vi "Settings Dialog.vi"(8 "error in (no error)":errorcluster, 11 "Feed Module Config in":T15={"GUID"="", "Drop Coords"={"Horizontal"=0, "Vertical"=0}, "Process Name"="", "Settings"={"Cycle Period"=500.0, "Ismatech"={"VISA resource name"="", "Simulated?"=TRUE, "Pump Number"=1.0, "Reverse?"=FALSE}, "Masterflex"={"VISA resource name"="", "Simulated?"=TRUE, "Pump Number"=1.0, "Reverse?"=FALSE}, "Mettler"={"VISA resource name"="", "Simulated?"=FALSE}, "Bronkhorst M13 Flow Meter"={"VISA resource name"="", "Simulated?"=TRUE}, "PID 2 Parameters"={"Input Device"=enum."Default", "Output Device"=enum."Default", "Setpoint"=0.0, "PID gains"={"proportional gain (Kc)"=1.0, "integral time (Ti, min)"=0.01, "derivative time (Td, min)"=0.0}}, "Manual Entry"=0.0, "Auto?"=TRUE, "output range"={"output high"=100.0, "output low"=0.0}, "Bronkhorst M14"={"VISA resource name"="", "Simulated?"=FALSE}, "Tacmina Settings"={"Analog DAQ Task"="", "Digital DAQ Task"=""}, "KNF SIMDOS Settings"={"VISA resource name"="", "Simulated?"=TRUE}, "ASIA Pump C"={"ASIA Pump #"=-1, "channel"=-1, "Simulated"=FALSE}, "VICI Settings"={"VISA resource name"="", "Simulated?"=TRUE, "Pump Letter"="", "Reverse?"=FALSE}, "FLOM Settings"={"VISA resource name"="", "Simulated?"=TRUE, "Pump Number"=0.0}, "SSI PR Settings"={"VISA resource name"="", "Simulated?"=FALSE}}, "Settings Load Count"=0, "OP Load Count"=0} {"Settings"."output range"."output low" min=0.0 max=100.0 format="%.2f"; "Settings"."output range"."output high" format="%.2f"; "Settings"."PID 2 Parameters"."PID gains"."derivative time (Td, min)" format="%.3f"; "Settings"."PID 2 Parameters"."PID gains"."integral time (Ti, min)" format="%.3f"; "Settings"."PID 2 Parameters"."PID gains"."proportional gain (Kc)" format="%.3f"; "Settings"."ASIA Pump C"."channel" min=0 max=1 step=1; "Settings"."Ismatech"."Pump Number" min=1.0 max=20.0 step=1.0; "Settings"."Masterflex"."Pump Number" min=1.0 max=20.0 step=1.0}) -> (0 "error out":errorcluster, 1 "Cancelled?":bool=TRUE, 2 "UI Refresh Needed?":bool, 3 "Feed Module Config out":T15={"GUID"="", "Drop Coords"={"Horizontal"=0, "Vertical"=0}, "Process Name"="", "Settings"={"Cycle Period"=500.0, "Ismatech"={"VISA resource name"="", "Simulated?"=TRUE, "Pump Number"=1.0, "Reverse?"=FALSE}, "Masterflex"={"VISA resource name"="", "Simulated?"=TRUE, "Pump Number"=1.0, "Reverse?"=FALSE}, "Mettler"={"VISA resource name"="", "Simulated?"=FALSE}, "Bronkhorst M13 Flow Meter"={"VISA resource name"="", "Simulated?"=TRUE}, "PID 2 Parameters"={"Input Device"=enum."Default", "Output Device"=enum."Default", "Setpoint"=0.0, "PID gains"={"proportional gain (Kc)"=1.0, "integral time (Ti, min)"=0.01, "derivative time (Td, min)"=0.0}}, "Manual Entry"=0.0, "Auto?"=TRUE, "output range"={"output high"=100.0, "output low"=0.0}, "Bronkhorst M14"={"VISA resource name"="", "Simulated?"=FALSE}, "Tacmina Settings"={"Analog DAQ Task"="", "Digital DAQ Task"=""}, "KNF SIMDOS Settings"={"VISA resource name"="", "Simulated?"=TRUE}, "ASIA Pump C"={"ASIA Pump #"=0, "channel"=0, "Simulated"=FALSE}, "VICI Settings"={"VISA resource name"="", "Simulated?"=TRUE, "Pump Letter"="", "Reverse?"=FALSE}, "FLOM Settings"={"VISA resource name"="", "Simulated?"=TRUE, "Pump Number"=0.0}, "SSI PR Settings"={"VISA resource name"="", "Simulated?"=FALSE}}, "Settings Load Count"=0, "OP Load Count"=0} {"Settings"."output range"."output low" min=0.0 max=100.0 format="%.2f"; "Settings"."output range"."output high" format="%.2f"; "Settings"."PID 2 Parameters"."PID gains"."derivative time (Td, min)" format="%.3f"; "Settings"."PID 2 Parameters"."PID gains"."integral time (Ti, min)" format="%.3f"; "Settings"."PID 2 Parameters"."PID gains"."proportional gain (Kc)" format="%.3f"; "Settings"."ASIA Pump C"."channel" min=0 max=1 step=1; "Settings"."Ismatech"."Pump Number" min=1.0 max=20.0 step=1.0; "Settings"."Masterflex"."Pump Number" min=1.0 max=20.0 step=1.0})   [LabVIEW 2018, in "Feed Module.lvlib" / "Settings.lvlib"]
doc: "Dialog for selecting user specified settings."
uses:
  Settings.lvlib
  Feed Module/Controls/Feed Module Config Cluster.ctl
  <vilib>/Utility/miscctls.llb/LVPoint32TypeDef.ctl
  Feed Module/Controls/Feed Module Settings Cluster.ctl
  Ismatec ISM 831C/Controls/Ismatech Settings Cluster.ctl
  Masterflex 7550-30/Controls/Settings Cluster.ctl
  Mettler Toledo/Controls/Settings Cluster.ctl
  Bronkhorst M13 Flow Meter/Settings Cluster.ctl
  Measure Instrument/PID 2 Parameters Cluster.ctl
  Measure Instrument/PID Input Enum.ctl
  Measure Instrument/PID 2 Output Enum.ctl
  Tacmina QI/Tacmina QI DAQ Setting.ctl
  KNF Pump/Settings Cluster plus SIMDOS.ctl
  ASIA Pump/Pump Settings.ctl
  VICI M50 Party Mode/Settings Cluster.ctl
  FLOM Pump/Settings Cluster.ctl
  SSI PR Class/SSI PR Settings Cluster.ctl
  Bronkhorst M14 Flow Meter/Settings Cluster.ctl
  Ismatec ISM 831C/Ismatec ISM 831C.lvlib
  Masterflex 7550-30/Masterflex 7550-30.lvlib
  Mettler Toledo/Mettler Toledo.lvlib
  Bronkhorst M13 Flow Meter/Bronkhorst M13 Flow Meter.lvlib
  Bronkhorst M14 Flow Meter/Bronkhorst M14 Flow Meter.lvlib
  KNF Pump/KNF SIMDOS.lvlib
  VICI M50 Party Mode/VICI M6 M50 Party Mode.lvlib
  FLOM Pump/FLOM Pump.lvlib
  ASIA Pump.lvlib
  SSI PR Class/SSI PR Pump.lvlib
  <vilib>/Utility/xml.llb/Write to XML File(string).vi
  Feed Module/Feed Module.lvlib
  Tacmina QI/Tacmina QI.lvlib
panel:
  in  "Module Name":string
  in  "Settings Dialog":T14={"Cycle Period"=500.0, "Ismatech"={"VISA resource name"="", "Simulated?"=FALSE, "Pump Number"=1.0, "Reverse?"=FALSE}, "Masterflex"={"VISA resource name"="", "Simulated?"=FALSE, "Pump Number"=1.0, "Reverse?"=FALSE}, "Mettler"={"VISA resource name"="", "Simulated?"=FALSE}, "Bronkhorst M13 Flow Meter"={"VISA resource name"="", "Simulated?"=FALSE}, "PID 2 Parameters"={"Input Device"=enum."Default", "Output Device"=enum."Default", "PID gains"={"proportional gain (Kc)"=1.0, "integral time (Ti, min)"=0.01, "derivative time (Td, min)"=0.0}}, "PID2 Range"={"output high"=100.0, "output low"=0.0}, "Bronkhorst M14 Settings"={"VISA resource name"="", "Simulated?"=FALSE}, "Tacmina Settings"={"Analog DAQ Task"="", "Digital DAQ Task"=""}, "KNF SIMDOS Settings"={"VISA resource name"="", "Simulated?"=FALSE}, "ASIA Pump C"={"ASIA Pump #"=-1, "channel"=-1, "Simulated"=FALSE}, "VICI M50 Settings"={"VISA resource name"="", "Simulated?"=FALSE, "Pump Letter"="", "Reverse?"=FALSE}, "FLOM Settings"={"VISA resource name"="", "Simulated?"=FALSE, "Pump Number"=1.0}, "SSI PR Settings"={"VISA resource name"="", "Simulated?"=FALSE}} {"ASIA Pump C"."channel" min=-1 max=1 step=1; "PID2 Range"."output low" min=0.0 max=100.0 format="%.2f"; "PID2 Range"."output high" format="%.2f"; "PID 2 Parameters"."PID gains"."derivative time (Td, min)" format="%.3f"; "PID 2 Parameters"."PID gains"."integral time (Ti, min)" format="%.3f"; "PID 2 Parameters"."PID gains"."proportional gain (Kc)" format="%.3f"; "Masterflex"."Pump Number" min=1.0 max=20.0 step=1.0; "Ismatech"."Pump Number" min=1.0 max=20.0 step=1.0}
  in  "Cancel Button":bool
  in  "OK Button":bool
  # "Non visible portion of dialog (needed for connector pane)."
  # "Output Instruments"
  # "Input Instruments"
  # "Output Instruments"
  # "Input Instruments"
  # "Output Instruments"
  # "Input Instruments"
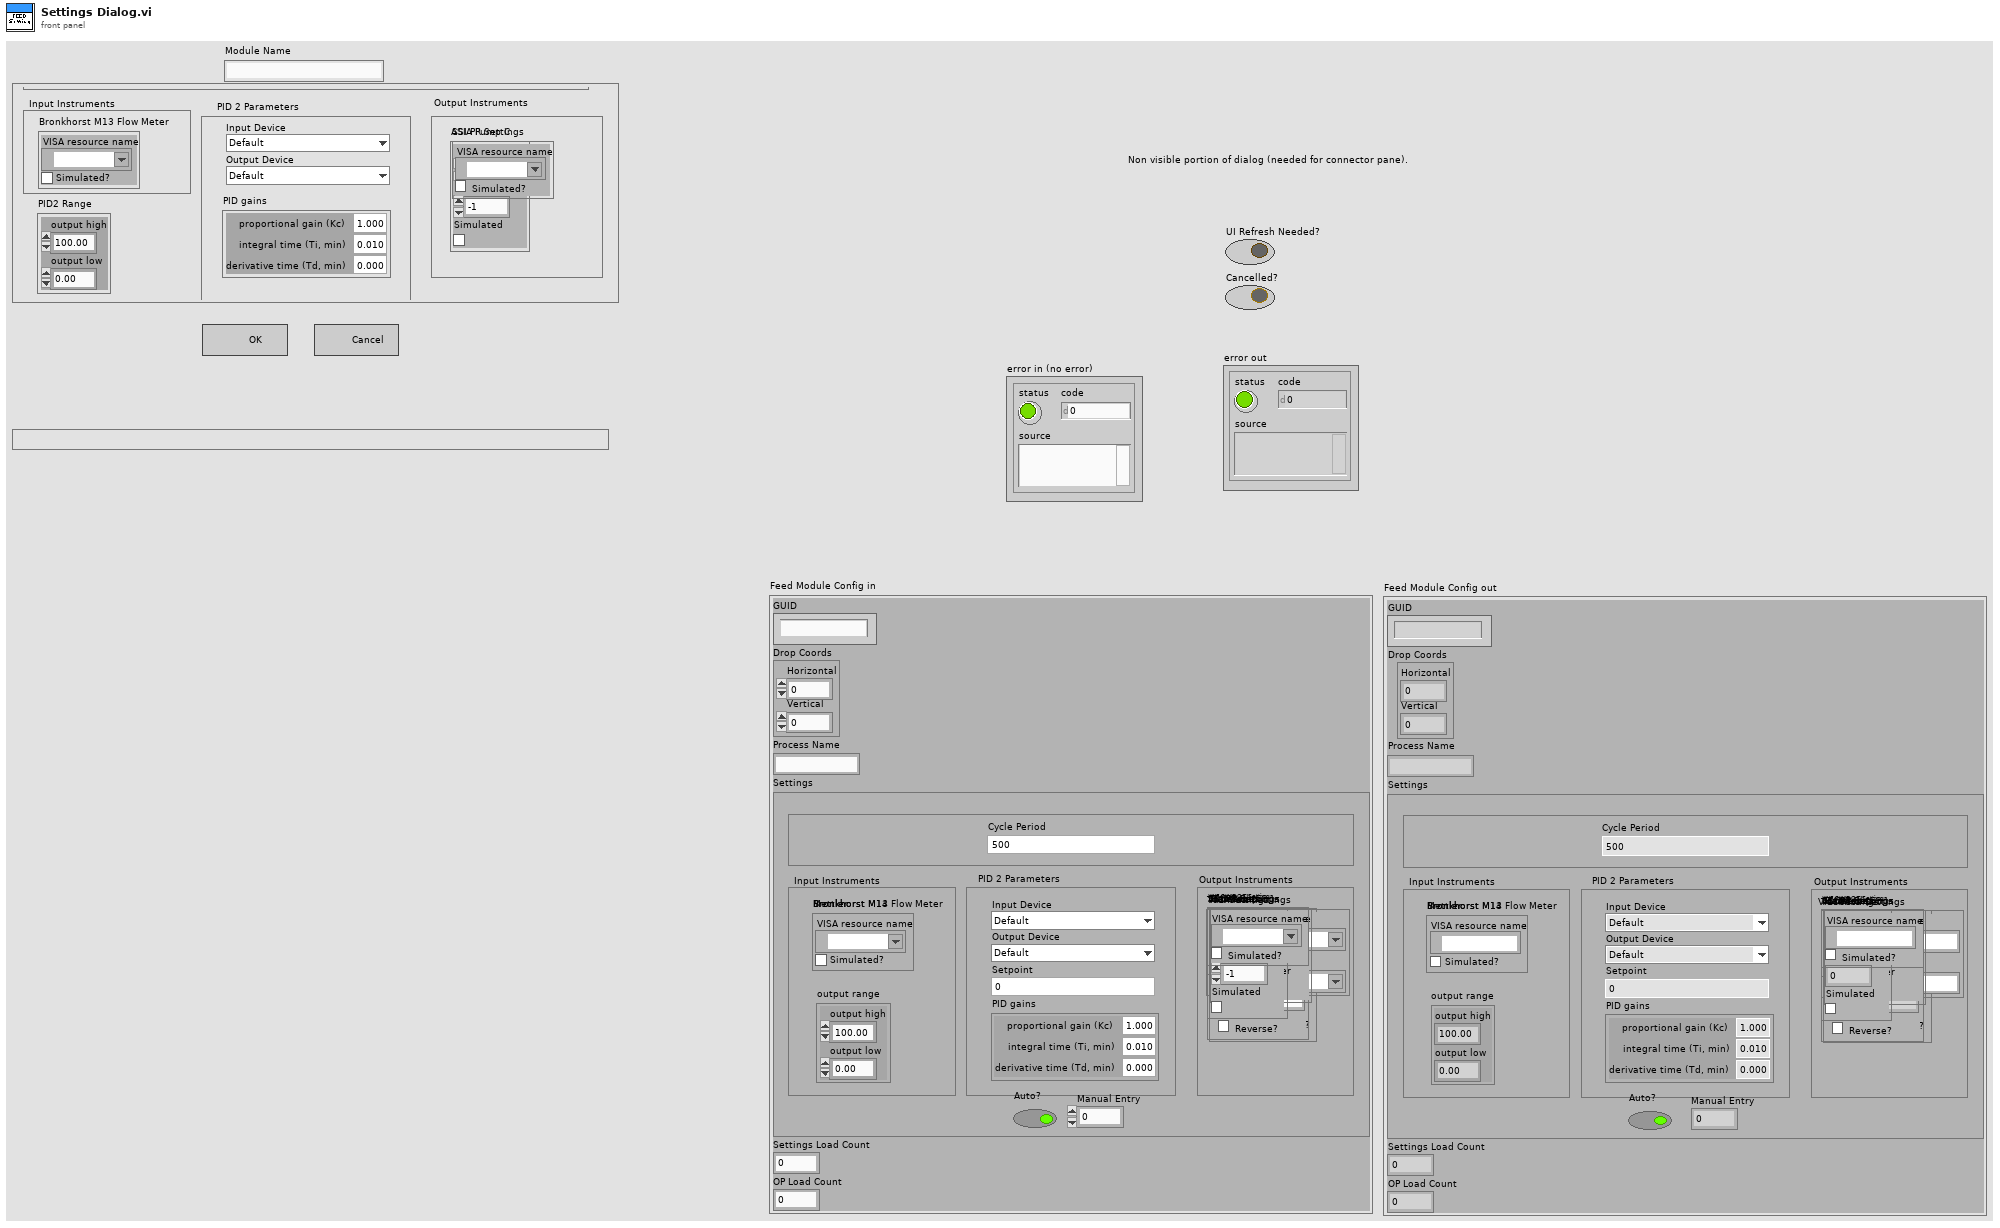
[diagram p1: front panel]
types:
  T1 = typedef "Ismatec ISM 831C.lvlib/Ismatech Settings Cluster.ctl" = cluster{"VISA resource name":refnum<visa-resource-name>, "Simulated?":bool, "Pump Number":dbl, "Reverse?":bool}
  T2 = typedef "Masterflex 7550-30.lvlib/Settings Cluster.ctl" = cluster{"VISA resource name":refnum<visa-resource-name>, "Simulated?":bool, "Pump Number":dbl, "Reverse?":bool}
  T3 = typedef "Mettler Toledo.lvlib/Settings Cluster.ctl" = cluster{"VISA resource name":refnum<visa-resource-name>, "Simulated?":bool}
  T4 = typedef "Bronkhorst M13 Flow Meter.lvlib/Settings Cluster.ctl" = cluster{"VISA resource name":refnum<visa-resource-name>, "Simulated?":bool}
  T5 = typedef "PID Input Enum.ctl" = enum16{"Default", "Bronkhorst M13", "Bronkhorst M14", "Scale Rate of Change"}
  T6 = typedef "PID 2 Output Enum.ctl" = enum16{"Default", "Ismatec ISM 831C", "Masterflex 7550-30", "VICI", "Tacmina QI", "KNF SIMDOS", "ASIA Type C", "FLOM UI-22-11", "SSI PR"}
  T7 = typedef "Bronkhorst M14 Flow Meter.lvlib/Settings Cluster.ctl" = cluster{"VISA resource name":refnum<visa-resource-name>, "Simulated?":bool}
  T8 = typedef "Tacmina QI.lvlib/Tacmina QI DAQ Setting.ctl" = cluster{"Analog DAQ Task":refnum<k21>, "Digital DAQ Task":refnum<k21>}
  T9 = typedef "KNF SIMDOS.lvlib/Settings Cluster plus SIMDOS.ctl" = cluster{"VISA resource name":refnum<visa-resource-name>, "Simulated?":bool}
  T10 = typedef "ASIA Pump.lvlib/Pump Settings.ctl" = cluster{"ASIA Pump #":i32, "channel":i32, "Simulated":bool}
  T11 = typedef "VICI M6 M50 Party Mode.lvlib/Settings Cluster.ctl" = cluster{"VISA resource name":refnum<visa-resource-name>, "Simulated?":bool, "Pump Letter":string, "Reverse?":bool}
  T12 = typedef "FLOM Pump.lvlib/Settings Cluster.ctl" = cluster{"VISA resource name":refnum<visa-resource-name>, "Simulated?":bool, "Pump Number":dbl}
  T13 = typedef "SSI PR Pump.lvlib/SSI PR Settings Cluster.ctl" = cluster{"VISA resource name":refnum<visa-resource-name>, "Simulated?":bool}
  T14 = cluster{"Cycle Period":dbl, "Ismatech":T1, "Masterflex":T2, "Mettler":T3, "Bronkhorst M13 Flow Meter":T4, "PID 2 Parameters":cluster{"Input Device":T5, "Output Device":T6, "PID gains":cluster{"proportional gain (Kc)":dbl, "integral time (Ti, min)":dbl, "derivative time (Td, min)":dbl}}, "PID2 Range":cluster{"output high":dbl, "output low":dbl}, "Bronkhorst M14 Settings":T7, "Tacmina Settings":T8, "KNF SIMDOS Settings":T9, "ASIA Pump C":T10, "VICI M50 Settings":T11, "FLOM Settings":T12, "SSI PR Settings":T13}
  T15 = typedef "Feed Module.lvlib/Feed Module Config Cluster.ctl" = cluster{"GUID":string, "Drop Coords":T16, "Process Name":string, "Settings":T17, "Settings Load Count":i32, "OP Load Count":i32}
  T16 = typedef "LVPoint32TypeDef.ctl" = cluster{"Horizontal":i32, "Vertical":i32}
  T17 = typedef "Feed Module.lvlib/Feed Module Settings Cluster.ctl" = cluster{"Cycle Period":dbl, "Ismatech":T1, "Masterflex":T2, "Mettler":T3, "Bronkhorst M13 Flow Meter":T4, "PID 2 Parameters":T18, "Manual Entry":dbl, "Auto?":bool, "output range":cluster{"output high":dbl, "output low":dbl}, "Bronkhorst M14":T3, "Tacmina Settings":T8, "KNF SIMDOS Settings":T9, "ASIA Pump C":T10, "VICI Settings":T11, "FLOM Settings":T12, "SSI PR Settings":T13}
  T18 = typedef "PID 2 Parameters Cluster.ctl" = cluster{"Input Device":T5, "Output Device":T6, "Setpoint":dbl, "PID gains":cluster{"proportional gain (Kc)":dbl, "integral time (Ti, min)":dbl, "derivative time (Td, min)":dbl}}
  T19 = enum8{"Enabled", "Disabled", "Disabled and Grayed Out"}
  T20 = cluster{"proportional gain (Kc)":dbl, "integral time (Ti, min)":dbl, "derivative time (Td, min)":dbl}
  T21 = cluster{"Input Device":T5, "Output Device":T6, "PID gains":cluster{"proportional gain (Kc)":dbl, "integral time (Ti, min)":dbl, "derivative time (Td, min)":dbl}}
  T22 = cluster{"Cycle Period":dbl, "Ismatech":T1, "Masterflex":T2, "Mettler":T3, "Bronkhorst M13 Flow Meter":T4, cluster{"Input Device":T5, "Output Device":T6, "PID gains":cluster{"proportional gain (Kc)":dbl, "integral time (Ti, min)":dbl, "derivative time (Td, min)":dbl}}, "output range":cluster{"output high":dbl, "output low":dbl}, "Bronkhorst M14":T3, "Tacmina Settings":T8, "KNF SIMDOS Settings":T9, "ASIA Pump C":T10, "VICI Settings":T11, "FLOM Settings":T12, "SSI PR Settings":T13}
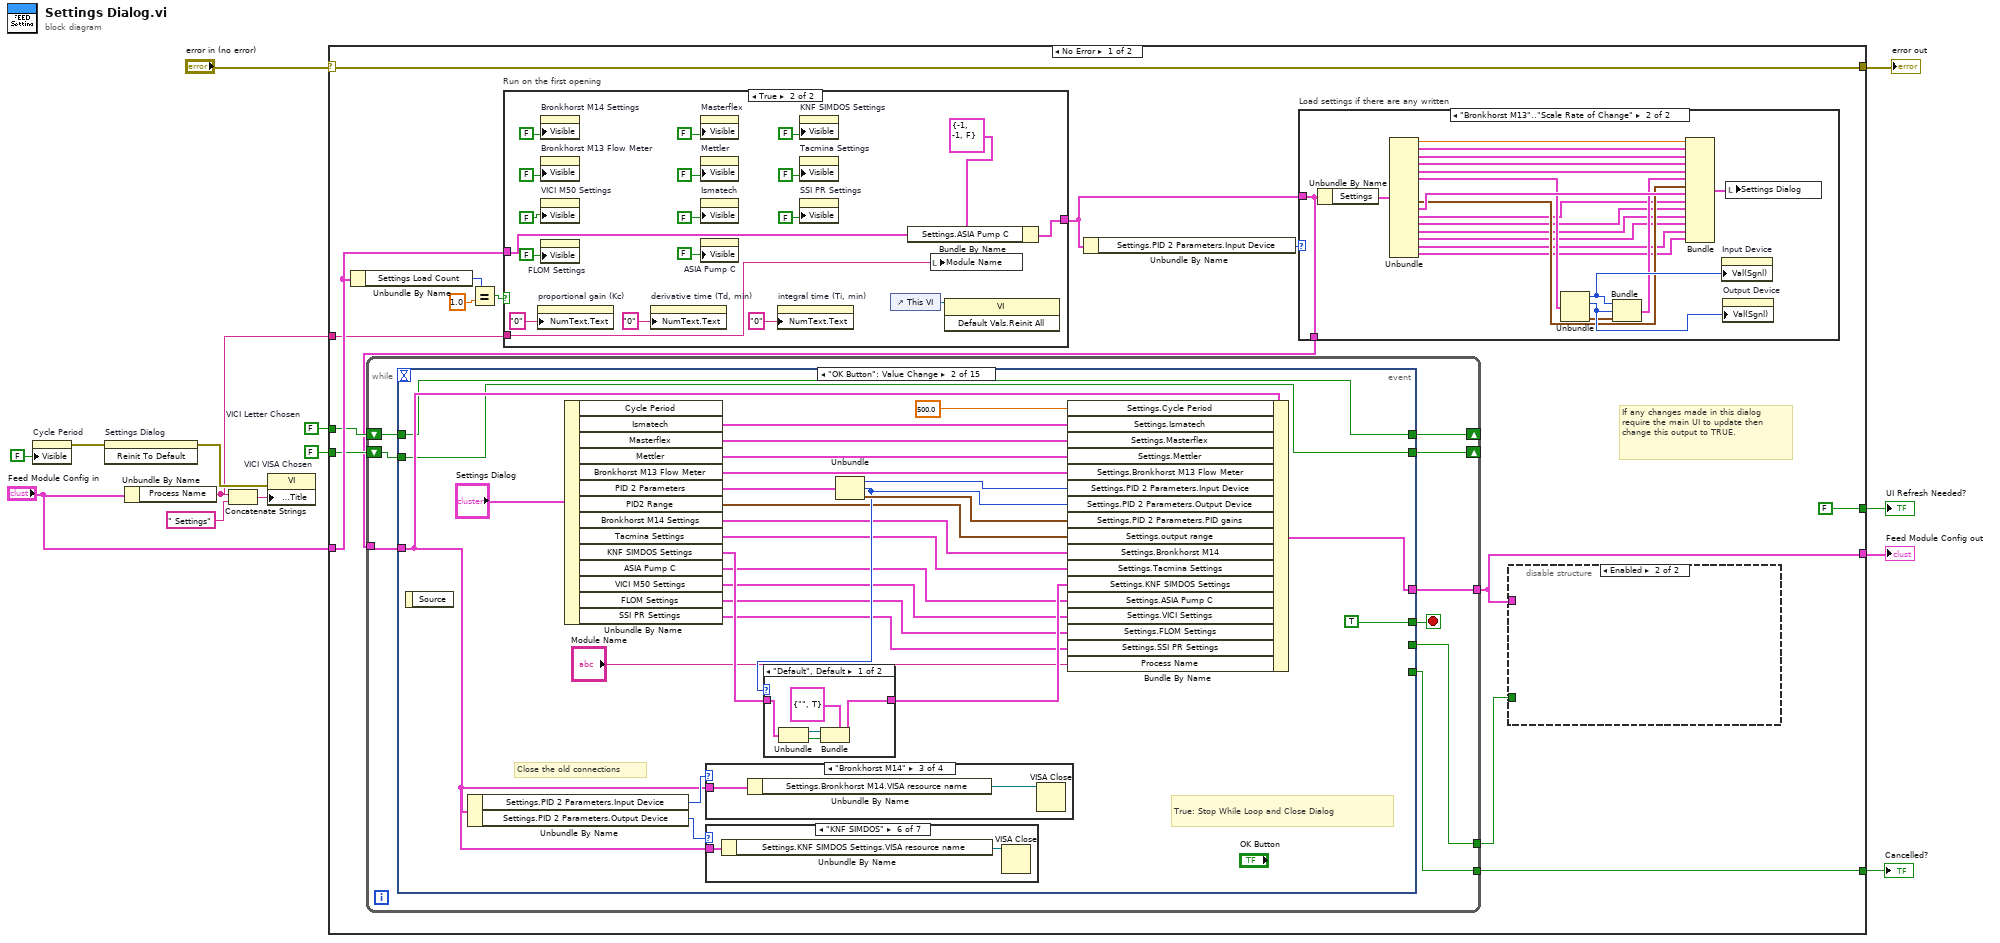
[diagram p0: block diagram]
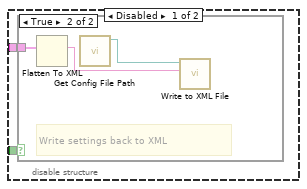
[diagram p2: hidden frame]
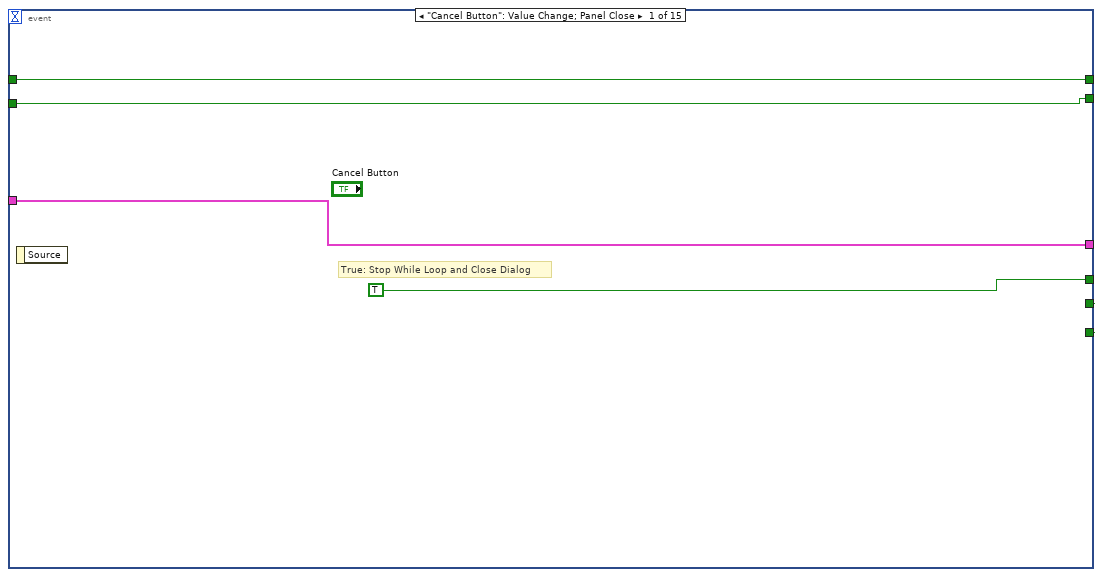
[diagram p6: hidden frame]
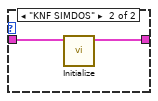
[diagram p7: hidden frame]
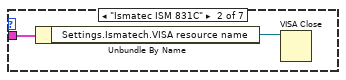
[diagram p9: hidden frame]
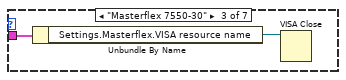
[diagram p10: hidden frame]
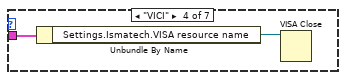
[diagram p11: hidden frame]
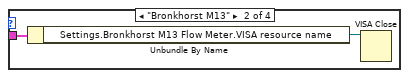
[diagram p15: hidden frame]
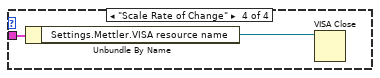
[diagram p16: hidden frame]
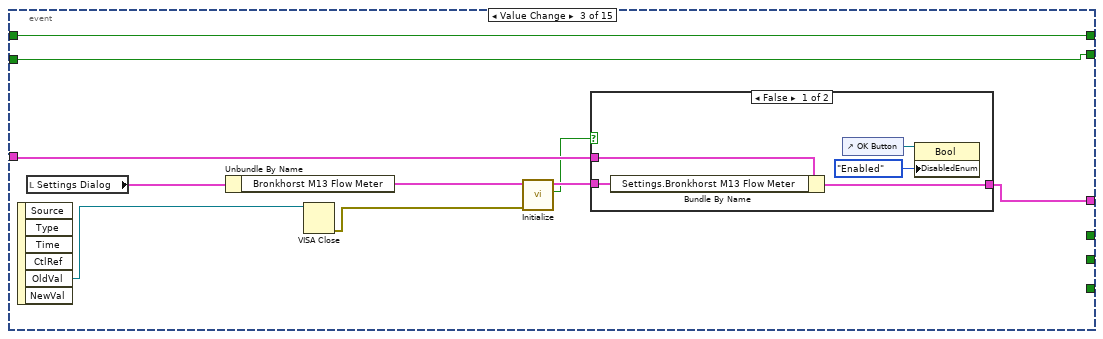
[diagram p17: hidden frame]
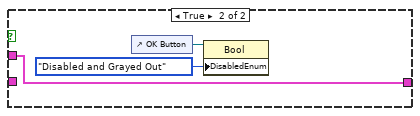
[diagram p18: hidden frame]
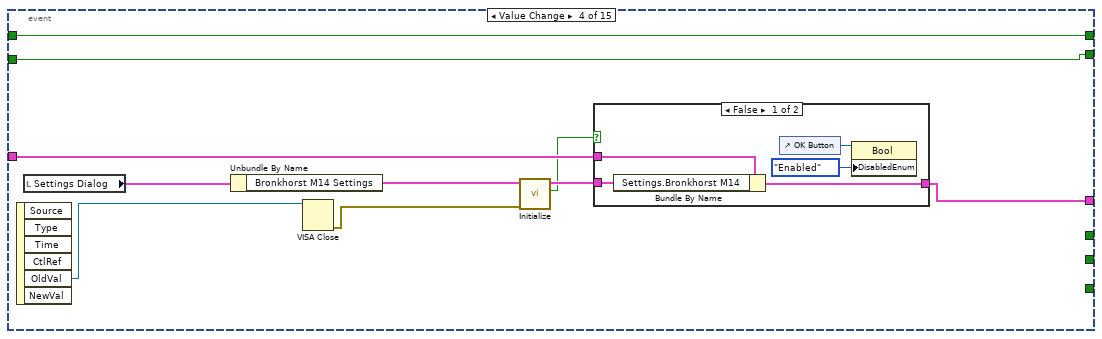
[diagram p19: hidden frame]
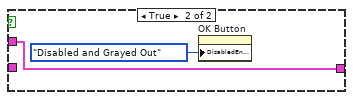
[diagram p20: hidden frame]
diagram:
  w5 = FALSE  # VICI VISA Chosen
  w6 = FALSE  # VICI Letter Chosen
  n1 = property on="Cycle Period" class="DigNum (strict)"("Visible"=FALSE) -> (error out=w3:errorcluster)  [unwired: 2 in, 1 out]
  n2 = invoke on="Settings Dialog" class="Clust (strict)" method="Reinit To Default"(error in=w3) -> (error out=w2:errorcluster)  [unwired: 2 in, 2 out]
  n3 = Unbundle By Name("Feed Module Config in") -> ("Process Name"=w1:string)
  n4 = Concatenate Strings(w1, " Settings" ("string")) -> (w8:string)
  n5 = property class="VI"(error in=w2, "Front Panel.Title"=w8) -> ()  [unwired: 1 in, 2 out]
  n6 = case shown="No Error" "error in (no error)" {
    selector: "error in (no error)" -> [w29 w507]
    tunnel: [w29 w507] -> w14
    tunnel: "Feed Module Config in" -> [w25 w506]
    tunnel: [w27 w506] -> w10
    tunnel: [FALSE ("UI Refresh Needed?") _] -> w13
    tunnel: [w26 TRUE ("UI Refresh Needed?")] -> w12
    tunnel: w6 -> [w18 _]
    tunnel: w5 -> [w17 _]
    tunnel: w1 -> [w15 _]
    frame No Error {
      # "If any changes made in this dialog require the main UI to update then change this output to TRUE."
      n7 = Unbundle By Name(w25) -> ("Settings Load Count"=w24:i32)
      n8 = Equal?(x=w24, y=1.0) -> (x = y?=w21:bool)
      n9 = case "Run on the first opening" shown="True" w21 {
        tunnel: w25 -> [w57 w62]
        tunnel: [w57 w61] -> w19
        tunnel: w15 -> [_ w58]
        frame False {
        }
        frame True {
          n10 = property on="proportional gain (Kc)" class="DigNum (strict)"("NumText.Text"="0" ("Numeric Text.Text")) -> ()  [unwired: 2 in, 2 out]
          n11 = property on="Bronkhorst M14 Settings" class="Clust (strict)"("Visible"=FALSE) -> ()  [unwired: 2 in, 2 out]
          n12 = property on="Bronkhorst M13 Flow Meter" class="Clust (strict)"("Visible"=FALSE) -> ()  [unwired: 2 in, 2 out]
          n13 = property on="VICI M50 Settings" class="Clust (strict)"("Visible"=FALSE) -> ()  [unwired: 2 in, 2 out]
          n14 = property on="FLOM Settings" class="Clust (strict)"("Visible"=FALSE) -> ()  [unwired: 2 in, 2 out]
          n15 = property on="derivative time (Td, min)" class="DigNum (strict)"("NumText.Text"="0" ("Numeric Text.Text")) -> ()  [unwired: 2 in, 2 out]
          n16 = property on="Masterflex" class="Clust (strict)"("Visible"=FALSE) -> ()  [unwired: 2 in, 2 out]
          n17 = property on="Mettler" class="Clust (strict)"("Visible"=FALSE) -> ()  [unwired: 2 in, 2 out]
          n18 = property on="Ismatech" class="Clust (strict)"("Visible"=FALSE) -> ()  [unwired: 2 in, 2 out]
          n19 = property on="ASIA Pump C" class="Clust (strict)"("Visible"=FALSE) -> ()  [unwired: 2 in, 2 out]
          n20 = property on="integral time (Ti, min)" class="DigNum (strict)"("NumText.Text"="0" ("Numeric Text.Text")) -> ()  [unwired: 2 in, 2 out]
          n21 = property on="KNF SIMDOS Settings" class="Clust (strict)"("Visible"=FALSE) -> ()  [unwired: 2 in, 2 out]
          n22 = property on="Tacmina Settings" class="Clust (strict)"("Visible"=FALSE) -> ()  [unwired: 2 in, 2 out]
          n23 = property on="SSI PR Settings" class="Clust (strict)"("Visible"=FALSE) -> ()  [unwired: 2 in, 2 out]
          n24 = control-ref of="This VI"() -> (w69:refnum<vi>)
          n25 = Bundle By Name(cluster=w62, "Settings.ASIA Pump C"=T10 {"ASIA Pump #"=-1, "channel"=-1, "Simulated"=FALSE}) -> (w61:T15)
          n26 = local write "Module Name"(w58) -> ()
          n27 = invoke class="VI" method="Default Vals.Reinit All"(reference=w69) -> ()  [unwired: 2 in, 3 out]
        }
      }
      n28 = Unbundle By Name(w19) -> ("Settings.PID 2 Parameters.Input Device"=w20:T5)
      n29 = case "Load settings if there are any written" shown="\"Bronkhorst M13\"..\"Scale Rate of Change\"" w20 {
        tunnel: w19 -> [w35 w38]
        tunnel: [w35 w38] -> w16
        frame "Default", Default {
        }
        frame "Bronkhorst M13".."Scale Rate of Change" {
          n30 = Unbundle By Name(w38) -> ("Settings"=w54:T17)
          n31 = Unbundle(w54) -> ("Cycle Period"=w55:dbl, "Ismatech"=w56:T1, "Masterflex"=w44:T2, "Mettler"=w45:T3, "Bronkhorst M13 Flow Meter"=w46:T4, "PID 2 Parameters"=w47:T18, "output range"=w49:cluster{"output high":dbl, "output low":dbl}, "Bronkhorst M14"=w51:T3, "Tacmina Settings"=w43:T8, "KNF SIMDOS Settings"=w42:T9, "ASIA Pump C"=w41:T10, "VICI Settings"=w40:T11, "FLOM Settings"=w39:T12, "SSI PR Settings"=w36:T13)  [unwired: 2 out]
          n32 = Unbundle(w47) -> ("Input Device"=w52:T5, "Output Device"=w53:T6, "PID gains"=w48:T20)  [unwired: 1 out]
          n33 = Bundle("Input Device"=w52, "Output Device"=w53, "PID gains"=w48) -> (w50:T21)  [unwired: 1 in]
          n34 = Bundle("Cycle Period"=w55, "Ismatech"=w56, "Masterflex"=w44, "Mettler"=w45, "Bronkhorst M13 Flow Meter"=w46, w50, "output range"=w49, "Bronkhorst M14"=w51, "Tacmina Settings"=w43, "KNF SIMDOS Settings"=w42, "ASIA Pump C"=w41, "VICI Settings"=w40, "FLOM Settings"=w39, "SSI PR Settings"=w36) -> (w37:T22)  [unwired: 1 in]
          n35 = property on="Input Device" class="Enum (strict)"("Val(Sgnl)"=w52) -> ()  [unwired: 2 in, 2 out]
          n36 = property on="Output Device" class="Enum (strict)"("Val(Sgnl)"=w53) -> ()  [unwired: 2 in, 2 out]
          n37 = local write "Settings Dialog"(w37) -> ()
        }
      }
      n38 = while {
        tunnel: [w85] -> w22
        tunnel: [w84] -> w27
        tunnel: [w82] -> w26
        shift-right: [w81] -> _
        shift-left: w18 -> [w80]
        shift-right: [w79] -> _
        shift-left: w17 -> [w78]
        tunnel: w16 -> [w77]
        stop <- w83 stop-if-true
        n39 = event shown="[1] \"OK Button\": Value Change" {
          selector: _ -> [_ _ _ _ _ _ _ _ _ _ _ _ _ _ _]
          dyn-events: _ -> [_ _ _ _ _ _ _ _ _ _ _ _ _ _ _]
          timeout: _ -> [_ _ _ _ _ _ _ _ _ _ _ _ _ _ _]
          tunnel: [w91 w118 w148 w166 w183 w209 w236 w254 w271 w291 w305 w346 w448 w465 w488] -> w84
          tunnel: w77 -> [w91 w106 w147 w165 w184 w210 w235 w255 w272 w292 w304 w346 w449 w464 w487]
          tunnel: [FALSE ("UI Refresh Needed?") FALSE ("UI Refresh Needed?") _ _ _ _ _ _ _ _ _ _ _ _ _] -> w85
          tunnel: [TRUE TRUE _ _ _ _ _ _ _ _ _ _ _ _ _] -> w83
          tunnel: [TRUE ("UI Refresh Needed?") FALSE ("UI Refresh Needed?") _ _ _ _ _ _ _ _ _ _ _ _ _] -> w82
          tunnel: [w87 w97 w143 w161 w182 w207 w230 w249 w268 w285 w303 w345 w446 TRUE w481] -> w81
          tunnel: w80 -> [w87 w97 w143 w161 w182 w207 w230 w249 w268 w285 w303 w345 w446 _ w481]
          tunnel: [w86 w96 w142 w160 w181 w206 w229 w248 w267 w284 w302 w344 w445 w460 TRUE] -> w79
          tunnel: w78 -> [w86 w96 w142 w160 w181 w206 w229 w248 w267 w284 w302 w344 w445 w460 _]
          event "Cancel Button": Value Change; Panel Close {
            # "True: Stop While Loop and Close Dialog"
            n40 = event-data() -> ()  [unwired: 1 in, 1 out]
          }
          event "OK Button": Value Change {
            # "Close the old connections"
            # "True: Stop While Loop and Close Dialog"
            n41 = event-data() -> ()  [unwired: 1 in, 1 out]
            n42 = Unbundle By Name(w106) -> ("Settings.PID 2 Parameters.Input Device"=w108:T5, "Settings.PID 2 Parameters.Output Device"=w107:T6)
            n43 = Unbundle By Name("Settings Dialog") -> ("Ismatech"=w116:T1, "Masterflex"=w115:T2, "Mettler"=w114:T3, "Bronkhorst M13 Flow Meter"=w113:T4, "PID 2 Parameters"=w112:T21, "PID2 Range"=w104:cluster{"output high":dbl, "output low":dbl}, "Bronkhorst M14 Settings"=w103:T7, "Tacmina Settings"=w102:T8, "KNF SIMDOS Settings"=w100:T9, "ASIA Pump C"=w99:T10, "VICI M50 Settings"=w98:T11, "FLOM Settings"=w95:T12, "SSI PR Settings"=w93:T13)  [unwired: 1 out]
            n44 = case shown="\"Bronkhorst M14\"" w108 {
              tunnel: w106 -> [_ w137 w138 w140]
              frame "Default", Default {
              }
              frame "Bronkhorst M13" {
                n45 = Unbundle By Name(w137) -> ("Settings.Bronkhorst M13 Flow Meter.VISA resource name"=w136:refnum<visa-resource-name>)
                n46 = VISA Close(VISA resource name=w136) -> ()  [unwired: 1 in, 1 out]
              }
              frame "Bronkhorst M14" {
                n47 = Unbundle By Name(w138) -> ("Settings.Bronkhorst M14.VISA resource name"=w139:refnum<visa-resource-name>)
                n48 = VISA Close(VISA resource name=w139) -> ()  [unwired: 1 in, 1 out]
              }
              frame "Scale Rate of Change" {
                n49 = Unbundle By Name(w140) -> ("Settings.Mettler.VISA resource name"=w141:refnum<visa-resource-name>)
                n50 = VISA Close(VISA resource name=w141) -> ()  [unwired: 1 in, 1 out]
              }
            }
            n51 = case shown="\"KNF SIMDOS\"" w107 {
              tunnel: w106 -> [_ w128 w130 w132 _ w135 _]
              frame "Default", Default {
              }
              frame "Ismatec ISM 831C" {
                n52 = Unbundle By Name(w128) -> ("Settings.Ismatech.VISA resource name"=w129:refnum<visa-resource-name>)
                n53 = VISA Close(VISA resource name=w129) -> ()  [unwired: 1 in, 1 out]
              }
              frame "Masterflex 7550-30" {
                n54 = Unbundle By Name(w130) -> ("Settings.Masterflex.VISA resource name"=w131:refnum<visa-resource-name>)
                n55 = VISA Close(VISA resource name=w131) -> ()  [unwired: 1 in, 1 out]
              }
              frame "VICI" {
                n56 = Unbundle By Name(w132) -> ("Settings.Ismatech.VISA resource name"=w133:refnum<visa-resource-name>)
                n57 = VISA Close(VISA resource name=w133) -> ()  [unwired: 1 in, 1 out]
              }
              frame "Tacmina QI" {
                # "No VISA to Close"
              }
              frame "KNF SIMDOS" {
                n58 = Unbundle By Name(w135) -> ("Settings.KNF SIMDOS Settings.VISA resource name"=w134:refnum<visa-resource-name>)
                n59 = VISA Close(VISA resource name=w134) -> ()  [unwired: 1 in, 1 out]
              }
              frame "ASIA Type C" {
                # "No VISA to Close"
              }
            }
            n60 = Unbundle(w112) -> ("Input Device"=w110:T5, "Output Device"=w105:T6, "PID gains"=w111:T20)
            n61 = case shown="\"Default\", Default" w105 {
              tunnel: w100 -> [w125 w126]
              tunnel: [w124 w127] -> w101
              frame "Default", Default {
                n62 = Unbundle(w125) -> ("VISA resource name"=w122:refnum<visa-resource-name>, "Simulated?"=w121:bool)
                n63 = Bundle(cluster=T9 {"VISA resource name"="", "Simulated?"=TRUE} ("KNF Settings"), "VISA resource name"=w122, "Simulated?"=w121) -> (w124:T9)
              }
              frame "KNF SIMDOS" {
                n64 = call "Initialize.vi"("KNF Settings"=w126) -> ("KNF Settings"=w127:T9)  [unwired: 7 in, 3 out]
              }
            }
            n65 = Bundle By Name(cluster=w106, "Settings.Cycle Period"=500.0, "Settings.Ismatech"=w116, "Settings.Masterflex"=w115, "Settings.Mettler"=w114, "Settings.Bronkhorst M13 Flow Meter"=w113, "Settings.PID 2 Parameters.Input Device"=w110, "Settings.PID 2 Parameters.Output Device"=w105, "Settings.PID 2 Parameters.PID gains"=w111, "Settings.output range"=w104, "Settings.Bronkhorst M14"=w103, "Settings.Tacmina Settings"=w102, "Settings.KNF SIMDOS Settings"=w101, "Settings.ASIA Pump C"=w99, "Settings.VICI Settings"=w98, "Settings.FLOM Settings"=w95, "Settings.SSI PR Settings"=w93, "Process Name"="Module Name") -> (w118:T15)
          }
          event Value Change {
            n66 = event-data() -> ("OldVal"=w145:refnum<visa-resource-name>)  [unwired: 1 in, 5 out]
            n67 = local read "Settings Dialog"() -> (w151:T14)
            n68 = Unbundle By Name(w151) -> ("Bronkhorst M13 Flow Meter"=w150:T4)
            n69 = VISA Close(VISA resource name=w145) -> (error out=w146:errorcluster)  [unwired: 1 in]
            n70 = call "Initialize.vi"("error in (no error)"=w146, "Bronkhorst Settings in"=w150) -> ("No Meter Connnected"=w144:bool, "Bronkhorst Settings out"=w149:T4)  [unwired: 7 in, 1 out]
            n71 = case shown="False" w144 {
              tunnel: w149 -> [w156 _]
              tunnel: [w155 w159] -> w148
              tunnel: w147 -> [w154 w159]
              frame False {
                n72 = Bundle By Name(cluster=w154, "Settings.Bronkhorst M13 Flow Meter"=w156) -> (w155:T15)
                n73 = control-ref of="OK Button"() -> (w152:refnum<vi>)
                n74 = property on="Property Node" class="Bool"(reference=w152, "DisabledEnum"=T19."Enabled" ("Disabled")) -> ()  [unwired: 1 in, 2 out]
              }
              frame True {
                n75 = control-ref of="OK Button"() -> (w157:refnum<vi>)
                n76 = property on="Property Node" class="Bool"(reference=w157, "DisabledEnum"=T19."Disabled and Grayed Out" ("Disabled")) -> ()  [unwired: 1 in, 2 out]
              }
            }
          }
          event Value Change {
            n77 = event-data() -> ("OldVal"=w163:refnum<visa-resource-name>)  [unwired: 1 in, 5 out]
            n78 = local read "Settings Dialog"() -> (w169:T14)
            n79 = Unbundle By Name(w169) -> ("Bronkhorst M14 Settings"=w168:T7)
            n80 = VISA Close(VISA resource name=w163) -> (error out=w164:errorcluster)  [unwired: 1 in]
            n81 = call "Initialize.vi"("error in (no error)"=w164, "Bronkhorst Settings in"=w168) -> ("No Meter Connected"=w162:bool, "Bronkhorst Settings out"=w167:T7)  [unwired: 7 in, 1 out]
            n82 = case shown="False" w162 {
              tunnel: w167 -> [w174 _]
              tunnel: [w173 w176] -> w166
              tunnel: w165 -> [w172 w176]
              frame False {
                n83 = Bundle By Name(cluster=w172, "Settings.Bronkhorst M14"=w174) -> (w173:T15)
                n84 = control-ref of="OK Button"() -> (w170:refnum<vi>)
                n85 = property on="Property Node" class="Bool"(reference=w170, "DisabledEnum"=T19."Enabled" ("Disabled")) -> ()  [unwired: 1 in, 2 out]
              }
              frame True {
                n86 = property on="OK Button" class="Bool"("DisabledEnum"=T19."Disabled and Grayed Out" ("Disabled")) -> ()  [unwired: 2 in, 2 out]
              }
            }
          }
          event Value Change {
            n87 = event-data() -> ()  [unwired: 1 in, 1 out]
            n88 = local read "Settings Dialog"() -> (w185:T14)
            n89 = Unbundle By Name(w185) -> ("FLOM Settings"=w178:T12)
            n90 = Unbundle By Name(w178) -> ("Pump Number"=w177:dbl)
            n91 = case shown="Default" w177 {
              tunnel: [w188 w191] -> w180
              tunnel: [w187 FALSE ("Initialized")] -> w179
              tunnel: w178 -> [w186 w191]
              frame Default {
                n92 = call "Initialize.vi"("FLOM Settings in"=w186) -> ("Initialized"=w187:bool, "FLOM Settings out"=w188:T12)  [unwired: 7 in, 2 out]
              }
              frame 0 {
                n93 = One Button Dialog(message="Choose a non-zero Pump Number") -> ()  [unwired: 1 in, 1 out]
              }
            }
            n94 = case shown="False" w179 {
              tunnel: w184 -> [w195 w200]
              tunnel: [w195 w199] -> w183
              tunnel: w180 -> [_ w198]
              frame False {
                n95 = control-ref of="OK Button"() -> (w193:refnum<vi>)
                n96 = property on="Property Node" class="Bool"(reference=w193, "DisabledEnum"=T19."Disabled and Grayed Out" ("Disabled")) -> ()  [unwired: 1 in, 2 out]
                n97 = One Button Dialog(message="No Pump Connected") -> ()  [unwired: 1 in, 1 out]
              }
              frame True {
                n98 = Bundle By Name(cluster=w200, "Settings.FLOM Settings"=w198) -> (w199:T15)
                n99 = control-ref of="OK Button"() -> (w196:refnum<vi>)
                n100 = property on="Property Node" class="Bool"(reference=w196, "DisabledEnum"=T19."Enabled" ("Disabled")) -> ()  [unwired: 1 in, 2 out]
              }
            }
          }
          event Value Change {
            n101 = event-data() -> ("OldVal"=w208:refnum<visa-resource-name>)  [unwired: 1 in]
            n102 = local read "Settings Dialog"() -> (w211:T14)
            n103 = Unbundle By Name(w211) -> ("FLOM Settings"=w202:T12)
            n104 = VISA Close(VISA resource name=w208) -> (error out=w205:errorcluster)  [unwired: 1 in]
            n105 = Unbundle By Name(w202) -> ("Pump Number"=w201:dbl)
            n106 = case shown="Default" w201 {
              tunnel: w205 -> [w215 _]
              tunnel: [w214 w218] -> w204
              tunnel: [w213 FALSE ("Initialized")] -> w203
              tunnel: w202 -> [w212 w218]
              frame Default {
                n107 = call "Initialize.vi"("error in (no error)"=w215, "FLOM Settings in"=w212) -> ("Initialized"=w213:bool, "FLOM Settings out"=w214:T12)  [unwired: 6 in, 2 out]
              }
              frame 0 {
                n108 = One Button Dialog(message="Choose a Pump Number") -> ()  [unwired: 1 in, 1 out]
              }
            }
            n109 = case shown="False" w203 {
              tunnel: w210 -> [w222 w227]
              tunnel: [w222 w226] -> w209
              tunnel: w204 -> [_ w225]
              frame False {
                n110 = control-ref of="OK Button"() -> (w220:refnum<vi>)
                n111 = One Button Dialog(message="No Pump Connected") -> ()  [unwired: 1 in, 1 out]
                n112 = property on="Property Node" class="Bool"(reference=w220, "DisabledEnum"=T19."Disabled and Grayed Out" ("Disabled")) -> ()  [unwired: 1 in, 2 out]
              }
              frame True {
                n113 = Bundle By Name(cluster=w227, "Settings.FLOM Settings"=w225) -> (w226:T15)
                n114 = control-ref of="OK Button"() -> (w223:refnum<vi>)
                n115 = property on="Property Node" class="Bool"(reference=w223, "DisabledEnum"=T19."Enabled" ("Disabled")) -> ()  [unwired: 1 in, 2 out]
              }
            }
          }
          event Value Change {
            n116 = event-data() -> ("OldVal"=w231:refnum<visa-resource-name>)  [unwired: 1 in, 5 out]
            n117 = local read "Settings Dialog"() -> (w234:T14)
            n118 = Unbundle By Name(w234) -> ("Ismatech"=w233:T1)
            n119 = VISA Close(VISA resource name=w231) -> (error out=w232:errorcluster)  [unwired: 1 in]
            n120 = call "Initialize.vi"("error in (no error)"=w232, "Ismatech Settings"=w233) -> ("Initialized"=w228:bool, "Ismatech Settings"=w237:T1)  [unwired: 6 in, 2 out]
            n121 = case shown="False" w228 {
              tunnel: w237 -> [_ w246]
              tunnel: [w241 w245] -> w236
              tunnel: w235 -> [w241 w244]
              frame False {
                n122 = control-ref of="OK Button"() -> (w239:refnum<vi>)
                n123 = property on="Property Node" class="Bool"(reference=w239, "DisabledEnum"=T19."Disabled and Grayed Out" ("Disabled")) -> ()  [unwired: 1 in, 2 out]
                n124 = One Button Dialog(message="No Pump Connected") -> ()  [unwired: 1 in, 1 out]
              }
              frame True {
                n125 = Bundle By Name(cluster=w244, "Settings.Ismatech"=w246) -> (w245:T15)
                n126 = control-ref of="OK Button"() -> (w242:refnum<vi>)
                n127 = property on="Property Node" class="Bool"(reference=w242, "DisabledEnum"=T19."Enabled" ("Disabled")) -> ()  [unwired: 1 in, 2 out]
              }
            }
          }
          event Value Change {
            n128 = event-data() -> ("OldVal"=w253:refnum<visa-resource-name>)  [unwired: 1 in, 5 out]
            n129 = local read "Settings Dialog"() -> (w256:T14)
            n130 = Unbundle By Name(w256) -> ("KNF SIMDOS Settings"=w251:T9)
            n131 = VISA Close(VISA resource name=w253) -> (error out=w252:errorcluster)  [unwired: 1 in]
            n132 = call "Initialize.vi"("error in (no error)"=w252, "KNF Settings"=w251) -> ("Initialized"=w247:bool, "KNF Settings"=w250:T9)  [unwired: 6 in, 2 out]
            n133 = case shown="False" w247 {
              tunnel: w255 -> [w260 w265]
              tunnel: [w260 w264] -> w254
              tunnel: w250 -> [_ w263]
              frame False {
                n134 = control-ref of="OK Button"() -> (w258:refnum<vi>)
                n135 = One Button Dialog(message="No Pump Connected") -> ()  [unwired: 1 in, 1 out]
                n136 = property on="Property Node" class="Bool"(reference=w258, "DisabledEnum"=T19."Disabled and Grayed Out" ("Disabled")) -> ()  [unwired: 1 in, 2 out]
              }
              frame True {
                n137 = Bundle By Name(cluster=w265, "Settings.KNF SIMDOS Settings"=w263) -> (w264:T15)
                n138 = control-ref of="OK Button"() -> (w261:refnum<vi>)
                n139 = property on="Property Node" class="Bool"(reference=w261, "DisabledEnum"=T19."Enabled" ("Disabled")) -> ()  [unwired: 1 in, 2 out]
              }
            }
          }
          event Value Change {
            n140 = event-data() -> ("OldVal"=w269:refnum<visa-resource-name>)  [unwired: 1 in, 5 out]
            n141 = local read "Settings Dialog"() -> (w273:T14)
            n142 = Unbundle By Name(w273) -> ("Masterflex"=w275:T2)
            n143 = VISA Close(VISA resource name=w269) -> (error out=w270:errorcluster)  [unwired: 1 in]
            n144 = call "Initialize.vi"("error in (no error)"=w270, "Masterflex Settings in"=w275) -> ("Initialized"=w266:bool, "Masterflex Settings out"=w274:T2)  [unwired: 6 in, 2 out]
            n145 = case shown="False" w266 {
              tunnel: w274 -> [_ w279]
              tunnel: w272 -> [w278 w283]
              tunnel: [w278 w282] -> w271
              frame False {
                n146 = control-ref of="OK Button"() -> (w276:refnum<vi>)
                n147 = property on="Property Node" class="Bool"(reference=w276, "DisabledEnum"=T19."Disabled and Grayed Out" ("Disabled")) -> ()  [unwired: 1 in, 2 out]
              }
              frame True {
                n148 = Bundle By Name(cluster=w283, "Settings.Masterflex"=w279) -> (w282:T15)
                n149 = control-ref of="OK Button"() -> (w280:refnum<vi>)
                n150 = property on="Property Node" class="Bool"(reference=w280, "DisabledEnum"=T19."Enabled" ("Disabled")) -> ()  [unwired: 1 in, 2 out]
              }
            }
          }
          event Value Change {
            n151 = event-data() -> ("OldVal"=w288:refnum<visa-resource-name>)  [unwired: 1 in, 5 out]
            n152 = local read "Settings Dialog"() -> (w293:T14)
            n153 = Unbundle By Name(w293) -> ("Mettler"=w290:T3)
            n154 = VISA Close(VISA resource name=w288) -> (error out=w287:errorcluster)  [unwired: 1 in]
            n155 = call "Initialize.vi"("error in (no error)"=w287, "Mettler Settings in"=w290) -> ("No Scale Connected"=w286:bool, "Mettler Settings out"=w289:T3)  [unwired: 7 in, 1 out]
            n156 = case shown="False" w286 {
              tunnel: w292 -> [w298 w301]
              tunnel: [w297 w301] -> w291
              tunnel: w289 -> [w296 _]
              frame False {
                n157 = Bundle By Name(cluster=w298, "Settings.Mettler"=w296) -> (w297:T15)
                n158 = control-ref of="OK Button"() -> (w294:refnum<vi>)
                n159 = property on="Property Node" class="Bool"(reference=w294, "DisabledEnum"=T19."Enabled" ("Disabled")) -> ()  [unwired: 1 in, 2 out]
              }
              frame True {
                n160 = control-ref of="OK Button"() -> (w299:refnum<vi>)
                n161 = property on="Property Node" class="Bool"(reference=w299, "DisabledEnum"=T19."Disabled and Grayed Out" ("Disabled")) -> ()  [unwired: 1 in, 2 out]
              }
            }
          }
          event Value Change {
            n162 = event-data() -> ("NewVal"=w306:T5)  [unwired: 1 in, 5 out]
            n163 = case "Show the correct settings" shown="\"Bronkhorst M13\"" w306 {
              tunnel: [w307 w317 w327 w338] -> w305
              tunnel: w304 -> [w307 w317 w327 w338]
              frame "Bronkhorst M13" {
                n164 = Unbundle By Name(w307) -> ("Settings.Bronkhorst M13 Flow Meter.VISA resource name"=w310:refnum<visa-resource-name>)
                n165 = Unbundle By Name(w307) -> ("Settings.PID 2 Parameters.Input Device"=w309:T5)
                n166 = property on="Mettler" class="Clust (strict)"("Visible"=FALSE) -> ()  [unwired: 2 in, 2 out]
                n167 = property on="Bronkhorst M13 Flow Meter" class="Clust (strict)"("Visible"=TRUE) -> ()  [unwired: 2 in, 2 out]
                n168 = property on="Bronkhorst M14 Settings" class="Clust (strict)"("Visible"=FALSE) -> ()  [unwired: 2 in, 2 out]
                n169 = case shown="\"Default\", Default" w309 {
                  frame "Default", Default {
                    n170 = property on="derivative time (Td, min)" class="DigNum (strict)"("NumText.Text"="0" ("Numeric Text.Text")) -> ()  [unwired: 2 in, 2 out]
                    n171 = property on="proportional gain (Kc)" class="DigNum (strict)"("NumText.Text"=".4" ("Numeric Text.Text")) -> ()  [unwired: 2 in, 2 out]
                    n172 = property on="integral time (Ti, min)" class="DigNum (strict)"("NumText.Text"="0.035" ("Numeric Text.Text")) -> ()  [unwired: 2 in, 2 out]
                  }
                  frame "Bronkhorst M13".."Scale Rate of Change" {
                  }
                }
                n173 = control-ref of="VISA resource name"() -> (w311:refnum<vi>)
                n174 = property on="Property Node" class="VISAName"(reference=w311, "Value"=w310) -> ()  [unwired: 1 in, 2 out]
              }
              frame "Bronkhorst M14" {
                n175 = Unbundle By Name(w317) -> ("Settings.PID 2 Parameters.Input Device"=w319:T5)
                n176 = Unbundle By Name(w317) -> ("Settings.Bronkhorst M14.VISA resource name"=w320:refnum<visa-resource-name>)
                n177 = property on="Bronkhorst M14 Settings" class="Clust (strict)"("Visible"=TRUE) -> ()  [unwired: 2 in, 2 out]
                n178 = property on="Mettler" class="Clust (strict)"("Visible"=FALSE) -> ()  [unwired: 2 in, 2 out]
                n179 = property on="Bronkhorst M13 Flow Meter" class="Clust (strict)"("Visible"=FALSE) -> ()  [unwired: 2 in, 2 out]
                n180 = control-ref of="VISA resource name"() -> (w321:refnum<vi>)
                n181 = case shown="\"Default\", Default" w319 {
                  frame "Default", Default {
                    n182 = property on="derivative time (Td, min)" class="DigNum (strict)"("NumText.Text"="0" ("Numeric Text.Text")) -> ()  [unwired: 2 in, 2 out]
                    n183 = property on="proportional gain (Kc)" class="DigNum (strict)"("NumText.Text"=".4" ("Numeric Text.Text")) -> ()  [unwired: 2 in, 2 out]
                    n184 = property on="integral time (Ti, min)" class="DigNum (strict)"("NumText.Text"="0.035" ("Numeric Text.Text")) -> ()  [unwired: 2 in, 2 out]
                  }
                  frame "Bronkhorst M13".."Scale Rate of Change" {
                  }
                }
                n185 = property on="Property Node" class="VISAName"(reference=w321, "Value"=w320) -> ()  [unwired: 1 in, 2 out]
              }
              frame "Scale Rate of Change" {
                n186 = Unbundle By Name(w327) -> ("Settings.PID 2 Parameters.Input Device"=w329:T5)
                n187 = property on="Bronkhorst M14 Settings" class="Clust (strict)"("Visible"=FALSE) -> ()  [unwired: 2 in, 2 out]
                n188 = property on="Mettler" class="Clust (strict)"("Visible"=TRUE) -> ()  [unwired: 2 in, 2 out]
                n189 = property on="Bronkhorst M13 Flow Meter" class="Clust (strict)"("Visible"=FALSE) -> ()  [unwired: 2 in, 2 out]
                n190 = Unbundle By Name(w327) -> ("Settings.Mettler.VISA resource name"=w331:refnum<visa-resource-name>)
                n191 = control-ref of="VISA resource name"() -> (w330:refnum<vi>)
                n192 = case shown="\"Default\", Default" w329 {
                  frame "Default", Default {
                    n193 = property on="derivative time (Td, min)" class="DigNum (strict)"("NumText.Text"="0" ("Numeric Text.Text")) -> ()  [unwired: 2 in, 2 out]
                    n194 = property on="proportional gain (Kc)" class="DigNum (strict)"("NumText.Text"=".4" ("Numeric Text.Text")) -> ()  [unwired: 2 in, 2 out]
                    n195 = property on="integral time (Ti, min)" class="DigNum (strict)"("NumText.Text"="0.035" ("Numeric Text.Text")) -> ()  [unwired: 2 in, 2 out]
                  }
                  frame "Bronkhorst M13".."Scale Rate of Change" {
                  }
                }
                n196 = property on="Property Node" class="VISAName"(reference=w330, "Value"=w331) -> ()  [unwired: 1 in, 2 out]
              }
              frame "Default", Default {
                n197 = property on="Bronkhorst M13 Flow Meter" class="Clust (strict)"("Visible"=FALSE) -> ()  [unwired: 2 in, 2 out]
                n198 = property on="Mettler" class="Clust (strict)"("Visible"=FALSE) -> ()  [unwired: 2 in, 2 out]
                n199 = property on="Bronkhorst M14 Settings" class="Clust (strict)"("Visible"=FALSE) -> ()  [unwired: 2 in, 2 out]
                n200 = property on="proportional gain (Kc)" class="DigNum (strict)"("NumText.Text"="0" ("Numeric Text.Text")) -> ()  [unwired: 2 in, 2 out]
                n201 = property on="integral time (Ti, min)" class="DigNum (strict)"("NumText.Text"="0" ("Numeric Text.Text")) -> ()  [unwired: 2 in, 2 out]
                n202 = property on="derivative time (Td, min)" class="DigNum (strict)"("NumText.Text"="0" ("Numeric Text.Text")) -> ()  [unwired: 2 in, 2 out]
              }
            }
          }
          event Value Change {
            n203 = event-data() -> ("NewVal"=w347:T6)  [unwired: 1 in]
            n204 = case "Show the correct settings" shown="\"ASIA Type C\"" w347 {
              tunnel: w346 -> [w354 w365 w376 w389 _ _ w413 w424 w431]
              frame "Ismatec ISM 831C" {
                n205 = property on="Ismatech" class="Clust (strict)"("Visible"=TRUE) -> ()  [unwired: 2 in, 2 out]
                n206 = property on="KNF SIMDOS Settings" class="Clust (strict)"("Visible"=FALSE) -> ()  [unwired: 2 in, 2 out]
                n207 = property on="Tacmina Settings" class="Clust (strict)"("Visible"=FALSE) -> ()  [unwired: 2 in, 2 out]
                n208 = Unbundle By Name(w354) -> ("Settings.Ismatech.VISA resource name"=w355:refnum<visa-resource-name>)
                n209 = property on="VICI M50 Settings" class="Clust (strict)"("Visible"=FALSE) -> ()  [unwired: 2 in, 2 out]
                n210 = property on="Masterflex" class="Clust (strict)"("Visible"=FALSE) -> ()  [unwired: 2 in, 2 out]
                n211 = property on="ASIA Pump C" class="Clust (strict)"("Visible"=FALSE) -> ()  [unwired: 2 in, 2 out]
                n212 = control-ref of="VISA resource name"() -> (w356:refnum<vi>)
                n213 = property on="SSI PR Settings" class="Clust (strict)"("Visible"=FALSE) -> ()  [unwired: 2 in, 2 out]
                n214 = property on="FLOM Settings" class="Clust (strict)"("Visible"=FALSE) -> ()  [unwired: 2 in, 2 out]
                n215 = property on="Property Node" class="VISAName"(reference=w356, "Value"=w355) -> ()  [unwired: 1 in, 2 out]
              }
              frame "FLOM UI-22-11" {
                n216 = property on="Tacmina Settings" class="Clust (strict)"("Visible"=FALSE) -> ()  [unwired: 2 in, 2 out]
                n217 = property on="Ismatech" class="Clust (strict)"("Visible"=FALSE) -> ()  [unwired: 2 in, 2 out]
                n218 = property on="KNF SIMDOS Settings" class="Clust (strict)"("Visible"=FALSE) -> ()  [unwired: 2 in, 2 out]
                n219 = Unbundle By Name(w365) -> ("Settings.FLOM Settings.VISA resource name"=w366:refnum<visa-resource-name>)
                n220 = property on="ASIA Pump C" class="Clust (strict)"("Visible"=FALSE) -> ()  [unwired: 2 in, 2 out]
                n221 = property on="VICI M50 Settings" class="Clust (strict)"("Visible"=FALSE) -> ()  [unwired: 2 in, 2 out]
                n222 = property on="Masterflex" class="Clust (strict)"("Visible"=FALSE) -> ()  [unwired: 2 in, 2 out]
                n223 = control-ref of="VISA resource name"() -> (w367:refnum<vi>)
                n224 = property on="FLOM Settings" class="Clust (strict)"("Visible"=TRUE) -> ()  [unwired: 2 in, 2 out]
                n225 = property on="SSI PR Settings" class="Clust (strict)"("Visible"=FALSE) -> ()  [unwired: 2 in, 2 out]
                n226 = property on="Property Node" class="VISAName"(reference=w367, "Value"=w366) -> ()  [unwired: 1 in, 2 out]
              }
              frame "Masterflex 7550-30" {
                n227 = property on="Masterflex" class="Clust (strict)"("Visible"=TRUE) -> ()  [unwired: 2 in, 2 out]
                n228 = property on="Tacmina Settings" class="Clust (strict)"("Visible"=FALSE) -> ()  [unwired: 2 in, 2 out]
                n229 = property on="KNF SIMDOS Settings" class="Clust (strict)"("Visible"=FALSE) -> ()  [unwired: 2 in, 2 out]
                n230 = Unbundle By Name(w376) -> ("Settings.Masterflex.VISA resource name"=w377:refnum<visa-resource-name>)
                n231 = property on="Ismatech" class="Clust (strict)"("Visible"=FALSE) -> ()  [unwired: 2 in, 2 out]
                n232 = property on="VICI M50 Settings" class="Clust (strict)"("Visible"=FALSE) -> ()  [unwired: 2 in, 2 out]
                n233 = control-ref of="VISA resource name"() -> (w378:refnum<vi>)
                n234 = property on="ASIA Pump C" class="Clust (strict)"("Visible"=FALSE) -> ()  [unwired: 2 in, 2 out]
                n235 = property on="SSI PR Settings" class="Clust (strict)"("Visible"=FALSE) -> ()  [unwired: 2 in, 2 out]
                n236 = property on="FLOM Settings" class="Clust (strict)"("Visible"=FALSE) -> ()  [unwired: 2 in, 2 out]
                n237 = property on="Property Node" class="VISAName"(reference=w378, "Value"=w377) -> ()  [unwired: 1 in, 2 out]
              }
              frame "VICI" {
                n238 = property on="KNF SIMDOS Settings" class="Clust (strict)"("Visible"=FALSE) -> ()  [unwired: 2 in, 2 out]
                n239 = property on="Masterflex" class="Clust (strict)"("Visible"=FALSE) -> ()  [unwired: 2 in, 2 out]
                n240 = property on="Tacmina Settings" class="Clust (strict)"("Visible"=FALSE) -> ()  [unwired: 2 in, 2 out]
                n241 = Unbundle By Name(w389) -> ("Settings.VICI Settings.VISA resource name"=w388:refnum<visa-resource-name>)
                n242 = property on="Ismatech" class="Clust (strict)"("Visible"=FALSE) -> ()  [unwired: 2 in, 2 out]
                n243 = property on="VICI M50 Settings" class="Clust (strict)"("Visible"=TRUE) -> ()  [unwired: 2 in, 2 out]
                n244 = property on="FLOM Settings" class="Clust (strict)"("Visible"=FALSE) -> ()  [unwired: 2 in, 2 out]
                n245 = property on="FLOM Settings" class="Clust (strict)"("Visible"=FALSE) -> ()  [unwired: 2 in, 2 out]
                n246 = property on="ASIA Pump C" class="Clust (strict)"("Visible"=FALSE) -> ()  [unwired: 2 in, 2 out]
                n247 = property on="VISA resource name" class="VISAName"("Value"=w388) -> ()  [unwired: 2 in, 2 out]
                n248 = property on="SSI PR Settings" class="Clust (strict)"("Visible"=FALSE) -> ()  [unwired: 2 in, 2 out]
              }
              frame "Default", Default {
                n249 = property on="VICI M50 Settings" class="Clust (strict)"("Visible"=FALSE) -> ()  [unwired: 2 in, 2 out]
                n250 = property on="KNF SIMDOS Settings" class="Clust (strict)"("Visible"=FALSE) -> ()  [unwired: 2 in, 2 out]
                n251 = property on="Tacmina Settings" class="Clust (strict)"("Visible"=FALSE) -> ()  [unwired: 2 in, 2 out]
                n252 = property on="Masterflex" class="Clust (strict)"("Visible"=FALSE) -> ()  [unwired: 2 in, 2 out]
                n253 = property on="Ismatech" class="Clust (strict)"("Visible"=FALSE) -> ()  [unwired: 2 in, 2 out]
                n254 = property on="FLOM Settings" class="Clust (strict)"("Visible"=FALSE) -> ()  [unwired: 2 in, 2 out]
                n255 = property on="ASIA Pump C" class="Clust (strict)"("Visible"=FALSE) -> ()  [unwired: 2 in, 2 out]
                n256 = property on="SSI PR Settings" class="Clust (strict)"("Visible"=FALSE) -> ()  [unwired: 2 in, 2 out]
              }
              frame "Tacmina QI" {
                n257 = property on="KNF SIMDOS Settings" class="Clust (strict)"("Visible"=FALSE) -> ()  [unwired: 2 in, 2 out]
                n258 = property on="Masterflex" class="Clust (strict)"("Visible"=FALSE) -> ()  [unwired: 2 in, 2 out]
                n259 = property on="Tacmina Settings" class="Clust (strict)"("Visible"=TRUE) -> ()  [unwired: 2 in, 2 out]
                n260 = property on="VICI M50 Settings" class="Clust (strict)"("Visible"=FALSE) -> ()  [unwired: 2 in, 2 out]
                n261 = property on="Ismatech" class="Clust (strict)"("Visible"=FALSE) -> ()  [unwired: 2 in, 2 out]
                n262 = property on="SSI PR Settings" class="Clust (strict)"("Visible"=FALSE) -> ()  [unwired: 2 in, 2 out]
                n263 = property on="FLOM Settings" class="Clust (strict)"("Visible"=FALSE) -> ()  [unwired: 2 in, 2 out]
                n264 = property on="ASIA Pump C" class="Clust (strict)"("Visible"=FALSE) -> ()  [unwired: 2 in, 2 out]
              }
              frame "KNF SIMDOS" {
                n265 = property on="Masterflex" class="Clust (strict)"("Visible"=FALSE) -> ()  [unwired: 2 in, 2 out]
                n266 = property on="Tacmina Settings" class="Clust (strict)"("Visible"=FALSE) -> ()  [unwired: 2 in, 2 out]
                n267 = property on="KNF SIMDOS Settings" class="Clust (strict)"("Visible"=TRUE) -> ()  [unwired: 2 in, 2 out]
                n268 = Unbundle By Name(w413) -> ("Settings.KNF SIMDOS Settings.VISA resource name"=w414:refnum<visa-resource-name>)
                n269 = property on="Ismatech" class="Clust (strict)"("Visible"=FALSE) -> ()  [unwired: 2 in, 2 out]
                n270 = property on="VICI M50 Settings" class="Clust (strict)"("Visible"=FALSE) -> ()  [unwired: 2 in, 2 out]
                n271 = property on="SSI PR Settings" class="Clust (strict)"("Visible"=FALSE) -> ()  [unwired: 2 in, 2 out]
                n272 = property on="ASIA Pump C" class="Clust (strict)"("Visible"=FALSE) -> ()  [unwired: 2 in, 2 out]
                n273 = property on="FLOM Settings" class="Clust (strict)"("Visible"=FALSE) -> ()  [unwired: 2 in, 2 out]
                n274 = property on="VISA resource name" class="VISAName"("Value"=w414) -> ()  [unwired: 2 in, 2 out]
              }
              frame "SSI PR" {
                n275 = property on="Masterflex" class="Clust (strict)"("Visible"=FALSE) -> ()  [unwired: 2 in, 2 out]
                n276 = property on="KNF SIMDOS Settings" class="Clust (strict)"("Visible"=FALSE) -> ()  [unwired: 2 in, 2 out]
                n277 = property on="Tacmina Settings" class="Clust (strict)"("Visible"=FALSE) -> ()  [unwired: 2 in, 2 out]
                n278 = Unbundle By Name(w424) -> ("Settings.SSI PR Settings.VISA resource name"=w418:refnum<visa-resource-name>)
                n279 = property on="VICI M50 Settings" class="Clust (strict)"("Visible"=FALSE) -> ()  [unwired: 2 in, 2 out]
                n280 = property on="Ismatech" class="Clust (strict)"("Visible"=FALSE) -> ()  [unwired: 2 in, 2 out]
                n281 = property on="SSI PR Settings" class="Clust (strict)"("Visible"=TRUE) -> ()  [unwired: 2 in, 2 out]
                n282 = property on="ASIA Pump C" class="Clust (strict)"("Visible"=FALSE) -> ()  [unwired: 2 in, 2 out]
                n283 = property on="FLOM Settings" class="Clust (strict)"("Visible"=FALSE) -> ()  [unwired: 2 in, 2 out]
                n284 = property on="VISA resource name" class="VISAName"("Value"=w418) -> ()  [unwired: 2 in, 2 out]
              }
              frame "ASIA Type C" {
                n285 = property on="Ismatech" class="Clust (strict)"("Visible"=FALSE) -> ()  [unwired: 2 in, 2 out]
                n286 = property on="KNF SIMDOS Settings" class="Clust (strict)"("Visible"=FALSE) -> ()  [unwired: 2 in, 2 out]
                n287 = Unbundle By Name(w431) -> ("Settings.ASIA Pump C.ASIA Pump #"=w434:i32)
                n288 = property on="VICI M50 Settings" class="Clust (strict)"("Visible"=FALSE) -> ()  [unwired: 2 in, 2 out]
                n289 = property on="Tacmina Settings" class="Clust (strict)"("Visible"=FALSE) -> ()  [unwired: 2 in, 2 out]
                n290 = Unbundle By Name(w431) -> ("Settings.ASIA Pump C.channel"=w433:i32)
                n291 = property on="ASIA Pump C" class="Clust (strict)"("Visible"=TRUE) -> ()  [unwired: 2 in, 2 out]
                n292 = property on="Masterflex" class="Clust (strict)"("Visible"=FALSE) -> ()  [unwired: 2 in, 2 out]
                n293 = control-ref of="channel"() -> (w432:refnum<vi>)
                n294 = control-ref of="ASIA Pump #"() -> (w435:refnum<vi>)
                n295 = property on="SSI PR Settings" class="Clust (strict)"("Visible"=FALSE) -> ()  [unwired: 2 in, 2 out]
                n296 = property on="FLOM Settings" class="Clust (strict)"("Visible"=FALSE) -> ()  [unwired: 2 in, 2 out]
                n297 = property on="Property Node" class="DigNum (strict)"(reference=w435, "Value"=w434) -> ()  [unwired: 1 in, 2 out]
                n298 = property on="Property Node" class="DigNum (strict)"(reference=w432, "Value"=w433) -> ()  [unwired: 1 in, 2 out]
              }
            }
          }
          event Value Change {
            n299 = event-data() -> ("OldVal"=w447:refnum<visa-resource-name>)  [unwired: 1 in, 5 out]
            n300 = local read "Settings Dialog"() -> (w450:T14)
            n301 = Unbundle By Name(w450) -> ("SSI PR Settings"=w444:T13)
            n302 = VISA Close(VISA resource name=w447) -> (error out=w443:errorcluster)  [unwired: 1 in]
            n303 = call "Initialize.vi"("error in (no error)"=w443, "SSI PR Settings In"=w444) -> ("Initialized"=w441:bool, "SSI PR Settings Out"=w442:T13)  [unwired: 6 in, 2 out]
            n304 = case shown="False" w441 {
              tunnel: w442 -> [_ w455]
              tunnel: w449 -> [w454 w459]
              tunnel: [w454 w458] -> w448
              frame False {
                n305 = control-ref of="OK Button"() -> (w452:refnum<vi>)
                n306 = property on="Property Node" class="Bool"(reference=w452, "DisabledEnum"=T19."Disabled and Grayed Out" ("Disabled")) -> ()  [unwired: 1 in, 2 out]
                n307 = One Button Dialog(message="No Pump Connected") -> ()  [unwired: 1 in, 1 out]
              }
              frame True {
                n308 = Bundle By Name(cluster=w459, "Settings.SSI PR Settings"=w455) -> (w458:T15)
                n309 = control-ref of="OK Button"() -> (w456:refnum<vi>)
                n310 = property on="Property Node" class="Bool"(reference=w456, "DisabledEnum"=T19."Enabled" ("Disabled")) -> ()  [unwired: 1 in, 2 out]
              }
            }
          }
          event Value Change {
            n311 = event-data() -> ()  [unwired: 1 in, 1 out]
            n312 = local read "Settings Dialog"() -> (w463:T14)
            n313 = Unbundle By Name(w463) -> ("VICI M50 Settings"=w462:T11)
            n314 = case shown="True" w460 {
              tunnel: [w466 w471] -> w465
              tunnel: w464 -> [w466 w470]
              tunnel: w462 -> [_ w468]
              frame False {
              }
              frame True {
                n315 = call "Initialize.vi"("VICI Settings"=w468) -> ("Initialized"=w467:bool, "VICI Settings"=w469:T11)  [unwired: 7 in, 2 out]
                n316 = case shown="False" w467 {
                  tunnel: [w475 w480] -> w471
                  tunnel: w470 -> [w475 w479]
                  tunnel: w469 -> [_ w476]
                  frame False {
                    n317 = control-ref of="OK Button"() -> (w473:refnum<vi>)
                    n318 = property on="Property Node" class="Bool"(reference=w473, "DisabledEnum"=T19."Disabled and Grayed Out" ("Disabled")) -> ()  [unwired: 1 in, 2 out]
                    n319 = One Button Dialog(message="No Pump Connected") -> ()  [unwired: 1 in, 1 out]
                  }
                  frame True {
                    n320 = Bundle By Name(cluster=w479, "Settings.VICI Settings"=w476) -> (w480:T15)
                    n321 = control-ref of="OK Button"() -> (w477:refnum<vi>)
                    n322 = property on="Property Node" class="Bool"(reference=w477, "DisabledEnum"=T19."Enabled" ("Disabled")) -> ()  [unwired: 1 in, 2 out]
                  }
                }
              }
            }
          }
          event Value Change {
            n323 = event-data() -> ("OldVal"=w483:refnum<visa-resource-name>)  [unwired: 1 in, 5 out]
            n324 = local read "Settings Dialog"() -> (w486:T14)
            n325 = Unbundle By Name(w486) -> ("VICI M50 Settings"=w485:T11)
            n326 = VISA Close(VISA resource name=w483) -> (error out=w484:errorcluster)  [unwired: 1 in]
            n327 = case shown="True" w481 {
              tunnel: [w489 w495] -> w488
              tunnel: w487 -> [w489 w494]
              tunnel: w485 -> [_ w492]
              tunnel: w484 -> [_ w491]
              frame False {
              }
              frame True {
                n328 = call "Initialize.vi"("error in (no error)"=w491, "VICI Settings"=w492) -> ("Initialized"=w490:bool, "VICI Settings"=w493:T11)  [unwired: 6 in, 2 out]
                n329 = case shown="False" w490 {
                  tunnel: [w499 w504] -> w495
                  tunnel: w494 -> [w499 w503]
                  tunnel: w493 -> [_ w500]
                  frame False {
                    n330 = control-ref of="OK Button"() -> (w497:refnum<vi>)
                    n331 = property on="Property Node" class="Bool"(reference=w497, "DisabledEnum"=T19."Disabled and Grayed Out" ("Disabled")) -> ()  [unwired: 1 in, 2 out]
                    n332 = One Button Dialog(message="No Pump Connected") -> ()  [unwired: 1 in, 1 out]
                  }
                  frame True {
                    n333 = Bundle By Name(cluster=w503, "Settings.VICI Settings"=w500) -> (w504:T15)
                    n334 = control-ref of="OK Button"() -> (w501:refnum<vi>)
                    n335 = property on="Property Node" class="Bool"(reference=w501, "DisabledEnum"=T19."Enabled" ("Disabled")) -> ()  [unwired: 1 in, 2 out]
                  }
                }
              }
            }
          }
        }
      }
      n336 = disable-structure shown="Enabled" {
        disable-tunnel: w27 -> [w31 _]
        disable-tunnel: w22 -> [w30 _]
        frame Disabled {
          n337 = case shown="True" w30 {
            tunnel: w31 -> [_ w33]
            frame False {
            }
            frame True {
              # "Write settings back to XML"
              n338 = Flatten To XML(anything=w33) -> (xml string=w32:string)
              n339 = call "Get Config File Path.vi"() -> ("XML File Path"=w34:path)  [unwired: 10 in, 1 out]
              n340 = call-poly <vilib>:"Write to XML File.vi"("XML Input"=w32, "XML File Path"=w34) -> ()  [unwired: 7 in, 3 out]
            }
          }
        }
        frame Enabled {
        }
      }
    }
    frame Error {
    }
  }
  "UI Refresh Needed?" <- w13
  "error out" <- w14
  "Feed Module Config out" <- w10
  "Cancelled?" <- w12
